vi "ziModSubscribe.vi"(7 "Error In":errorcluster, 9 "Path":string="/", 10 "ModHandle In":T1 {"ModHandle" format="0x%08x"; "Conn" format="0x%08x"}) -> (0 "Error Out":errorcluster, 3 "ModHandle Out":T1 {"ModHandle" format="0x%08x"; "Conn" format="0x%08x"})   [LabVIEW 2018, in "Zurich Instruments LabOne.lvlib"]
doc: "Subscribes the module to a node, which will be measured as soon as the module is executed."
uses:
  Zurich Instruments LabOne.lvlib
  <instrlib>/Zurich Instruments LabOne/Private/ziLV64.framework
  ziTypeModHandle.ctl
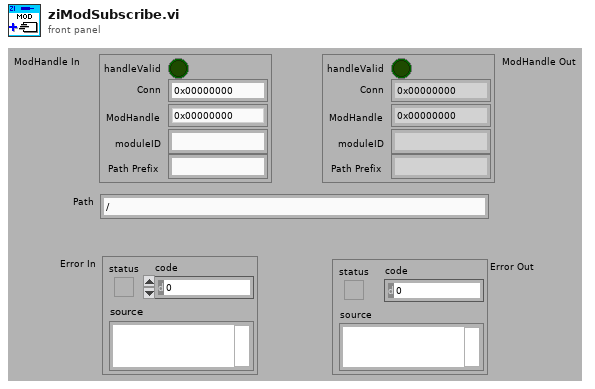
[diagram p1: front panel]
types:
  T1 = typedef "Zurich Instruments LabOne.lvlib/ziTypeModHandle.ctl" = cluster{"handleValid":bool, "Conn":u64, "ModHandle":u64, "moduleID":string, "Path Prefix":string}
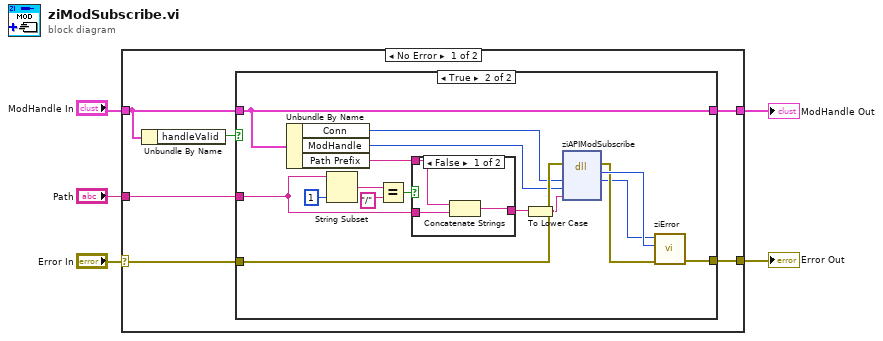
[diagram p0: block diagram]
diagram:
  n1 = case shown="No Error" "Error In" {
    selector: "Error In" -> [w9 w35]
    tunnel: "ModHandle In" -> [w7 w34]
    tunnel: [w11 w34] -> w2
    tunnel: [w10 w35] -> w5
    tunnel: "Path" -> [w6 _]
    frame No Error {
      n2 = Unbundle By Name(w7) -> ("handleValid"=w8:bool)
      n3 = case shown="True" w8 {
        tunnel: w7 -> [w13 w17]
        tunnel: [w13 w17] -> w11
        tunnel: w9 -> [w12 w29]
        tunnel: [w12 w24] -> w10
        tunnel: w6 -> [_ w19]
        frame False {
        }
        frame True {
          n4 = Unbundle By Name(w17) -> ("Conn"=w28:u64, "ModHandle"=w27:u64, "Path Prefix"=w18:string)
          n5 = String Subset(string=w19, length (rest)=1 ("length (rest)")) -> (substring=w22:string)  [unwired: 1 out]
          n6 = Equal?(x=w22, y="/") -> (x = y?=w20:bool)
          n7 = case shown="False" w20 {
            tunnel: w18 -> [w30 _]
            tunnel: [w32 w33] -> w16
            tunnel: w19 -> [w31 w33]
            frame False {
              n8 = Concatenate Strings(w30, w31) -> (w32:string)
            }
            frame True {
            }
          }
          n9 = To Lower Case(string=w16) -> (all lower case string=w15:string)
          n10 = dll-call lib="Applications/National Instruments/LabVIEW 2019 64-bit/instr.lib/Zurich Instruments LabOne/Private/ziLV*.*" fn="ziAPIModSubscribe"(error in=w29, "conn"=w28, "ModHandle"=w27, "Path"=w15) -> (error out=w25:errorcluster, "return type"=w26:u32, "conn"=w14:u64)  [unwired: 4 in, 1 out]
          n11 = call "ziError.vi"("Conn"=w14, "ziErrorCode"=w26, "Error In"=w25) -> ("Error Out"=w24:errorcluster)  [unwired: 3 in]
        }
      }
    }
    frame Error {
    }
  }
  "Error Out" <- w5
  "ModHandle Out" <- w2
